vi "Advance past Array.vi"(7 "JSON":string, 9 "Offset":i32) -> (1 "Offset past Array":i32, 2 "Empty Array":bool, 3 "State":T1, 6 "Array Start":i32)   [LabVIEW 2017, in "JSONtext.lvlib"]
uses:
  JSONtext.lvlib
  Parsing State.ctl
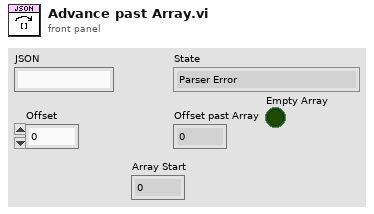
[diagram p1: front panel]
types:
  T1 = typedef "JSONtext.lvlib/Parsing State.ctl" = enum16{"Parser Error", "Object", "Array", "String", "Number/Other", "Leading Whitespace", "Object end", "Array end", "Value end"}
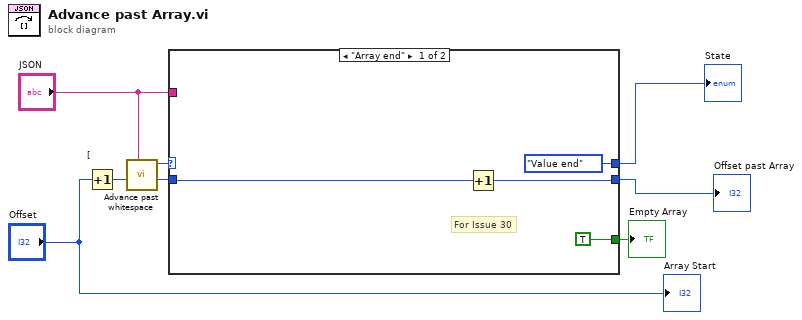
[diagram p0: block diagram]
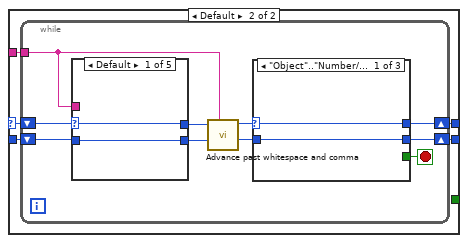
[diagram p2: hidden frame]
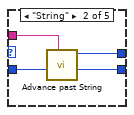
[diagram p3: hidden frame]
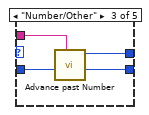
[diagram p4: hidden frame]
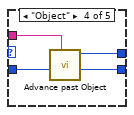
[diagram p5: hidden frame]
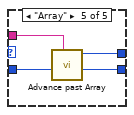
[diagram p6: hidden frame]
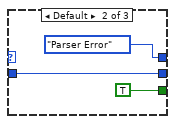
[diagram p7: hidden frame]
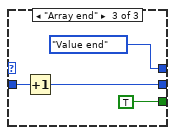
[diagram p8: hidden frame]
diagram:
  n1 = Increment "["(x="Offset") -> (x+1=w4:i32)
  n2 = call "Advance past whitespace.vi"("JSON"="JSON", "Offset"=w4) -> ("Offset of first non-whitespace"=w3:i32, "Parser State"=w5:T1)  [unwired: 8 in]
  n3 = case shown="\"Array end\"" w5 {
    selector: w5 -> [_ w15]
    tunnel: [w11 w17] -> w8
    tunnel: [Parsing_State."Value end" ("Parser State") w16] -> w6
    tunnel: w3 -> [w10 w14]
    tunnel: "JSON" -> [_ w13]
    tunnel: [TRUE _] -> w1
    frame "Array end" {
      # "For Issue 30"
      n4 = Increment(x=w10) -> (x+1=w11:i32)
    }
    frame Default {
      n5 = while {
        tunnel: w13 -> [w20]
        shift-right: [w25] -> w17
        shift-left: w14 -> [w18]
        shift-right: [w21] -> w16
        shift-left: w15 -> [w19]
        stop <- w24 stop-if-true
        n6 = case shown="Default" w19 {
          selector: w19 -> [w29 _ _ _ _]
          tunnel: w18 -> [w28 w31 w35 w41 w45]
          tunnel: [w29 w33 w37 w40 w43] -> w23
          tunnel: [w28 w32 w36 w39 w44] -> w22
          tunnel: w20 -> [_ w30 w34 w38 w42]
          frame Default {
          }
          frame "String" {
            n7 = call "Advance past String.vi"("JSON"=w30, "Offset"=w31) -> ("Offset past match"=w32:i32, "State"=w33:T1)  [unwired: 7 in, 1 out]
          }
          frame "Number/Other" {
            n8 = call "Advance past Number.vi"("JSON"=w34, "Offset (0)"=w35) -> ("Offset past match"=w36:i32, "Parser State"=w37:T1)  [unwired: 6 in, 2 out]
          }
          frame "Object" {
            n9 = call "Advance past Object.vi"("JSON"=w38, "Offset"=w41) -> ("Offset past Object"=w39:i32, "State"=w40:T1)  [unwired: 7 in, 1 out]
          }
          frame "Array" {
            n10 = call "Advance past Array.vi"("JSON"=w42, "Offset"=w45) -> ("Offset past Array"=w44:i32, "State"=w43:T1)  [unwired: 6 in, 2 out]
          }
        }
        n11 = call "Advance past whitespace and comma.vi"("JSON"=w20, "Offset"=w22, "State in"=w23) -> ("Offset past match"=w27:i32, "State"=w26:T1)  [unwired: 7 in]
        n12 = case shown="\"Object\"..\"Number/Other\"" w26 {
          selector: w26 -> [w46 _ _]
          tunnel: [_ TRUE TRUE] -> w24
          tunnel: w27 -> [w47 w49 w53]
          tunnel: [w47 w49 w52] -> w25
          tunnel: [w46 Parsing_State."Parser Error" Parsing_State."Value end"] -> w21
          frame "Object".."Number/Other" {
          }
          frame Default {
          }
          frame "Array end" {
            n13 = Increment(x=w53) -> (x+1=w52:i32)
          }
        }
      }
    }
  }
  "State" <- w6
  "Offset past Array" <- w8
  "Empty Array" <- w1
  "Array Start" <- "Offset"
